vi "Test Delete Tree.vi"(8 "Error In":errorcluster, 11 "Server Connection Information":T1) -> (0 "Error Out":errorcluster)   [LabVIEW 2017, in "Unit Tests.lvlib"]
uses:
  Unit Tests.lvlib
  source/Browser Core/Server Classes/UA Server/Server Connection Information.ctl
  source/Browser Core/Server Classes/UA Server/UA Server.lvclass
  source/Browser Core/Server Classes/UA Server/UA Server.lvclass/UA Server.ctl
  <vilib>/addons/_JKI Toolkits/Caraya/classes/Test/Test.lvclass
  <vilib>/addons/_JKI Toolkits/Caraya/classes/Assert/Assert.lvclass
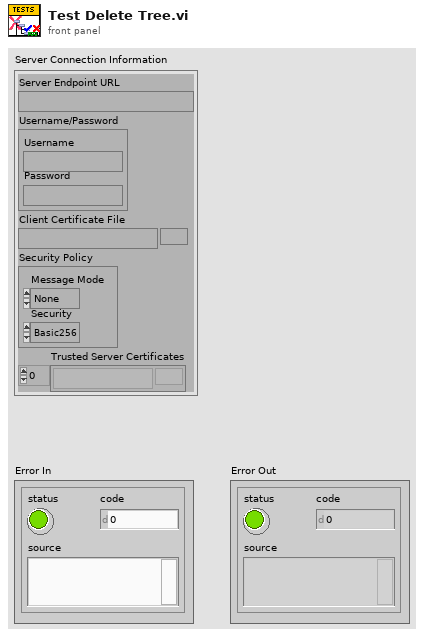
[diagram p1: front panel]
types:
  T1 = typedef "Browser Core.lvlib/UA Server.lvclass/Server Connection Information.ctl" = cluster{"Server Endpoint URL":string, "Username/Password":cluster{"Username":string, "Password":string}, "Client Certificate File":path, "Security Policy":cluster{"Message Mode":enum16{"None", "Sign", "Sign and Encrypt"}, "Security":enum16{"Basic256", "Basic128Rsa15"}}, "Trusted Server Certificates":path[]}
  T2 = cluster{"Message Mode":enum16{"None", "Sign", "Sign and Encrypt"}, "Security":enum16{"Basic256", "Basic128Rsa15"}}
  T3 = typedef "OPC UA Client Refnum.ctl" = refnum<k21>
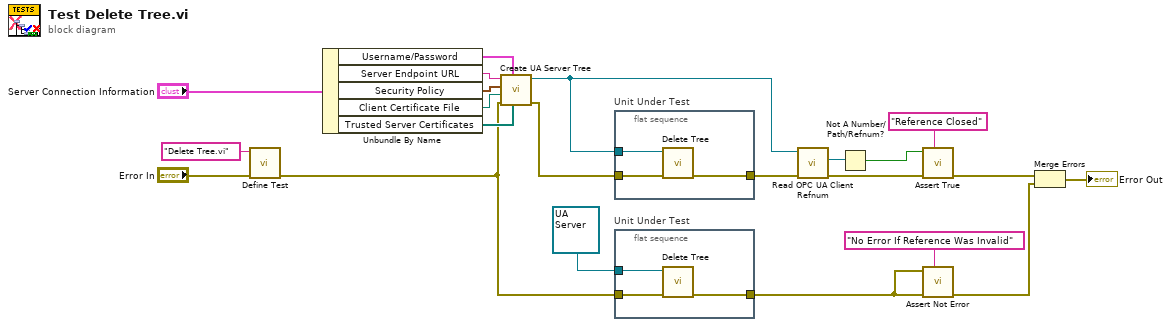
[diagram p0: block diagram]
diagram:
  n1 = call <vilib>:"Define Test.vi"("error in (no error)"="Error In", "Label (VI Title)"="Delete Tree.vi") -> ("error out"=w6:errorcluster)  [unwired: 9 in]
  n2 = Unbundle By Name("Server Connection Information") -> ("Username/Password"=w21:cluster{"Username":string, "Password":string}, "Server Endpoint URL"=w20:string, "Security Policy"=w19:T2, "Client Certificate File"=w18:path, "Trusted Server Certificates"=w17:path[])
  n3 = call "Create UA Server Tree.vi"("Trusted Server Certificates"=w17, "Username/Password"=w21, "Error In"=w6, "Client Certificate File"=w18, "Security Policy"=w19, "Server Endpoint URL"=w20) -> ("Error Out"=w16:errorcluster, "UA Server Tree"=w14:refnum<class "UA Server.lvclass">)  [unwired: 4 in]
  n4 = flat-sequence "Unit Under Test" {
    tunnel: w16 -> [w25]
    tunnel: [w24] -> w15
    tunnel: w14 -> [w23]
    frame #0 {
      n5 = call-dynamic "Delete Tree.vi"("error in (no error)"=w25, "UA Server in"=w23) -> ("error out"=w24:errorcluster)  [unwired: 9 in]
    }
  }
  n6 = flat-sequence "Unit Under Test" {
    tunnel: w6 -> [w28]
    tunnel: [w27] -> w2
    tunnel: refnum<class "UA Server.lvclass"> refnum ("UA Server in") -> [w26]
    frame #0 {
      n7 = call-dynamic "Delete Tree.vi"("error in (no error)"=w28, "UA Server in"=w26) -> ("error out"=w27:errorcluster)  [unwired: 9 in]
    }
  }
  n8 = call "Read OPC UA Client Refnum.vi"("error in (no error)"=w15, "UA Server in"=w14) -> ("error out"=w11:errorcluster, "OPC UA client refnum"=w9:T3)  [unwired: 7 in, 1 out]
  n9 = Not A Number/Path/Refnum?(number/path/refnum=w9) -> (NaN/Path/Refnum?=w8:bool)
  n10 = call <vilib>:"Assert True.vi"("Label"="Reference Closed", "error in (no error)"=w11, "True?"=w8) -> ("error out"=w10:errorcluster)  [unwired: 8 in]
  n11 = call <vilib>:"Assert Not Error.vi"("Label"="No Error If Reference Was Invalid", "error in (no error)"=w2, "Not Error?"=w2) -> ("error out"=w3:errorcluster)  [unwired: 8 in]
  n12 = Merge Errors(w10, w3) -> (→"Error Out":errorcluster)
